vi "BusEvents.vi"(0 "EventArray":variant[](array[variant]), 7 "Error in":errorcluster[](array[cluster]), 10 "ModuleList":string[](array[string])) -> (20 "SyncEvts":T3, 21 "FGenEvts":T4, 22 "DigitizerEvts":T5, 23 "AnalysisBroadcastEvents":T2, 24 "SensorBdcstEvents":T1, 27 "Error out":errorcluster[](array[cluster]))   [LabVIEW 2014]
uses:
  Modules/Digitizer/DigitizerModule/Protected/Broadcasts/clBroadcastEvents.ctl
  Modules/Digitizer/DigitizerModule/Protected/clEventType.ctl
  Modules/FGen/FgenModule/Protected/Broadcasts/clBroadcastEvents.ctl
  Modules/FGen/FgenModule/Protected/clEventType.ctl
  Modules/Sync/SyncModule/Protected/Broadcasts/clBroadcastEvents.ctl
  Modules/Sync/SyncModule/Protected/clEventType.ctl
  Modules/Analysis/AnalysisModule/Protected/Broadcasts/clBroadcastEvents.ctl
  Modules/Analysis/AnalysisModule/Protected/clEventType.ctl
  Modules/Sensor/SensorModule/Protected/Broadcasts/clBroadcastEvents.ctl
  Modules/Sensor/SensorModule/Protected/clEventType.ctl
  <vilib>/Utility/error.llb/Error Cluster From Error Code.vi
  <vilib>/ErrorRing/Error Ring.xnode
  Modules/Digitizer/DigitizerModule/DigitizerModule.lvlib
  Modules/FGen/FgenModule/FgenModule.lvlib
  Modules/Sync/SyncModule/SyncModule.lvlib
  <userlib>/NIST/NISTErrorLib/NISTErrorLib.lvlib
  Modules/Analysis/AnalysisModule/AnalysisModule.lvlib
  Modules/Sensor/SensorModule/SensorModule.lvlib
panel:
  # "If you want to add other Broadcast Events, open this typedef, copy an existing event and rename it to your event name.\n\nNext create an \"arg\" typedef for the  data and put it into PublicAPI/Arguments/Broadcasts\n\nAfter that, you will need to create a new roadcast vi in Protected/Broadcast.  Look at DidInit.vi or the reportError.vi as examples."
  # "If you want to add other Broadcast Events, open this typedef, copy an existing event and rename it to your event name.\n\nNext create an \"arg\" typedef for the  data and put it into PublicAPI/Arguments/Broadcasts\n\nAfter that, you will need to create a new roadcast vi in Protected/Broadcast.  Look at DidInit.vi or the reportError.vi as examples."
  # "If you want to add other Broadcast Events, open this typedef, copy an existing event and rename it to your event name.\n\nNext create an \"arg\" typedef for the  data and put it into PublicAPI/Arguments/Broadcasts\n\nAfter that, you will need to create a new roadcast vi in Protected/Broadcast.  Look at DidInit.vi or the reportError.vi as examples."
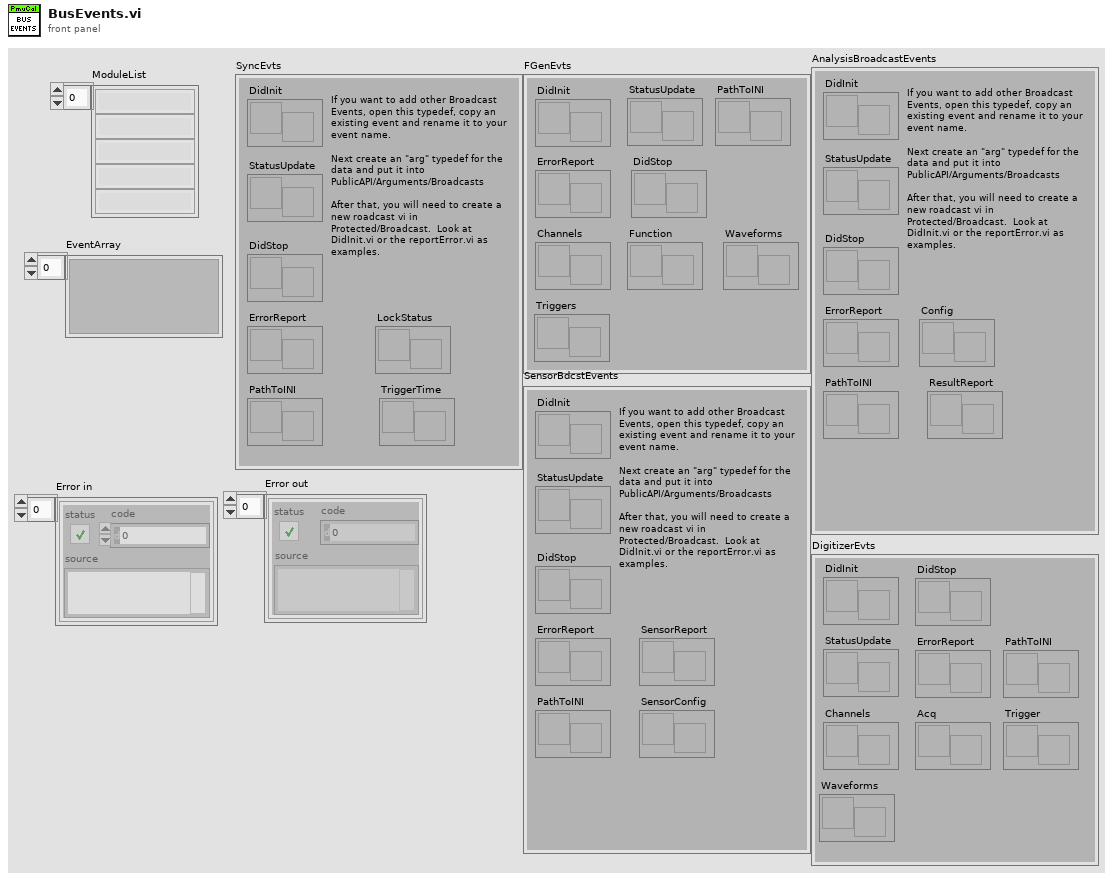
[diagram p1: front panel]
types:
  T1 = typedef "SensorModule.lvlib/clBroadcastEvents.ctl" = cluster{"DidInit":refnum<user-event>, "StatusUpdate":refnum<user-event>, "ErrorReport":refnum<user-event>, "DidStop":refnum<user-event>, "PathToINI":refnum<user-event>, "SensorReport":refnum<user-event>, "SensorConfig":refnum<user-event>}
  T2 = typedef "AnalysisModule.lvlib/clBroadcastEvents.ctl" = cluster{"DidInit":refnum<user-event>, "StatusUpdate":refnum<user-event>, "ErrorReport":refnum<user-event>, "DidStop":refnum<user-event>, "PathToINI":refnum<user-event>, "Config":refnum<user-event>, "ResultReport":refnum<user-event>}
  T3 = typedef "SyncModule.lvlib/clBroadcastEvents.ctl" = cluster{"DidInit":refnum<user-event>, "StatusUpdate":refnum<user-event>, "ErrorReport":refnum<user-event>, "DidStop":refnum<user-event>, "PathToINI":refnum<user-event>, "TriggerTime":refnum<user-event>, "LockStatus":refnum<user-event>}
  T4 = typedef "FgenModule.lvlib/clBroadcastEvents.ctl" = cluster{"DidInit":refnum<user-event>, "StatusUpdate":refnum<user-event>, "ErrorReport":refnum<user-event>, "DidStop":refnum<user-event>, "PathToINI":refnum<user-event>, "Channels":refnum<user-event>, "Function":refnum<user-event>, "Waveforms":refnum<user-event>, "Triggers":refnum<user-event>}
  T5 = typedef "DigitizerModule.lvlib/clBroadcastEvents.ctl" = cluster{"DidInit":refnum<user-event>, "StatusUpdate":refnum<user-event>, "ErrorReport":refnum<user-event>, "DidStop":refnum<user-event>, "PathToINI":refnum<user-event>, "Channels":refnum<user-event>, "Acq":refnum<user-event>, "Trigger":refnum<user-event>, "Waveforms":refnum<user-event>}
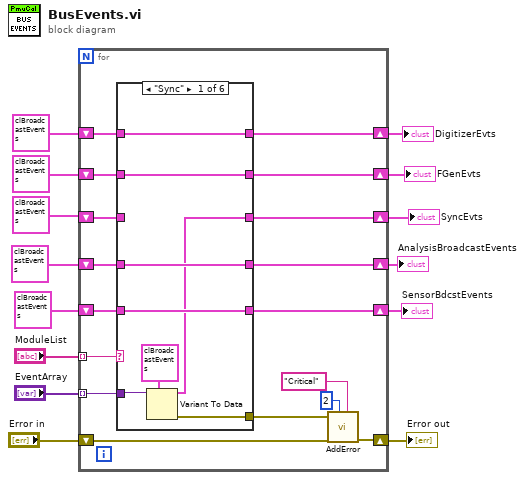
[diagram p0: block diagram]
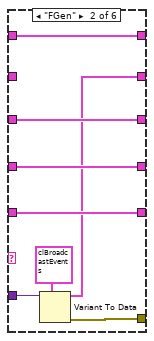
[diagram p2: hidden frame]
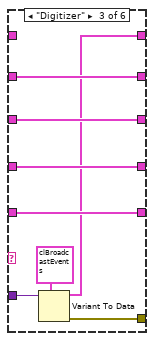
[diagram p3: hidden frame]
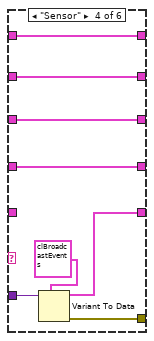
[diagram p4: hidden frame]
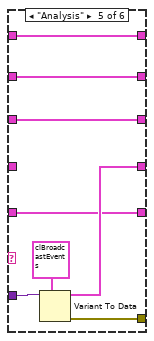
[diagram p5: hidden frame]
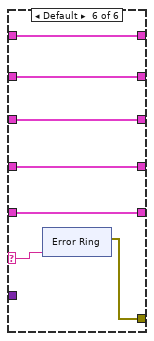
[diagram p6: hidden frame]
diagram:
  n1 = for {
    tunnel: "ModuleList" -> [w27] mode=indexing
    tunnel: "EventArray" -> [w26] mode=indexing
    shift-right: [w29] -> w5
    shift-left: "Error in" -> [w28]
    shift-right: [w23] -> w8
    shift-left: T5 {"DidInit"=refnum, "StatusUpdate"=refnum, "ErrorReport"=refnum, "DidStop"=refnum, "PathToINI"=refnum, "Channels"=refnum, "Acq"=refnum, "Trigger"=refnum, "Waveforms"=refnum} ("clBroadcastEvents") -> [w24]
    shift-right: [w19] -> w6
    shift-left: T3 {"DidInit"=refnum, "StatusUpdate"=refnum, "ErrorReport"=refnum, "DidStop"=refnum, "PathToINI"=refnum, "TriggerTime"=refnum, "LockStatus"=refnum} ("SyncBroadcastEvents") -> [w21]
    shift-right: [w20] -> w7
    shift-left: T4 {"DidInit"=refnum, "StatusUpdate"=refnum, "ErrorReport"=refnum, "DidStop"=refnum, "PathToINI"=refnum, "Channels"=refnum, "Function"=refnum, "Waveforms"=refnum, "Triggers"=refnum} ("clBroadcastEvents") -> [w22]
    shift-right: [w17] -> w3
    shift-left: T2 {"DidInit"=refnum, "StatusUpdate"=refnum, "ErrorReport"=refnum, "DidStop"=refnum, "PathToINI"=refnum, "Config"=refnum, "ResultReport"=refnum} ("AnalysisBroadcastEvents") -> [w18]
    shift-right: [w15] -> w1
    shift-left: T1 {"DidInit"=refnum, "StatusUpdate"=refnum, "ErrorReport"=refnum, "DidStop"=refnum, "PathToINI"=refnum, "SensorReport"=refnum, "SensorConfig"=refnum} ("SensorBdcstEvents") -> [w16]
    n2 = case shown="\"Sync\"" w27 {
      selector: w27 -> [_ _ _ _ _ w75]
      tunnel: w26 -> [w38 w47 w51 w60 w71 _]
      tunnel: [w37 w46 w55 w63 w70 w74] -> w25
      tunnel: w24 -> [w35 w44 _ w58 w67 w78]
      tunnel: [w35 w44 w48 w58 w67 w78] -> w23
      tunnel: w22 -> [w36 _ w53 w62 w66 w77]
      tunnel: [w36 w40 w53 w62 w66 w77] -> w20
      tunnel: w21 -> [_ w43 w52 w61 w65 w76]
      tunnel: [w32 w43 w52 w61 w65 w76] -> w19
      tunnel: [w34 w42 w50 w59 w68 w73] -> w17
      tunnel: w18 -> [w34 w42 w50 w59 _ w73]
      tunnel: [w33 w41 w49 w56 w64 w72] -> w15
      tunnel: w16 -> [w33 w41 w49 _ w64 w72]
      frame "Sync" {
        n3 = Variant To Data(type=T3 {"DidInit"=refnum, "StatusUpdate"=refnum, "ErrorReport"=refnum, "DidStop"=refnum, "PathToINI"=refnum, "TriggerTime"=refnum, "LockStatus"=refnum} ("SyncBroadcastEvents"), Variant=w38) -> (data=w32:T3, error out=w37:errorcluster)  [unwired: 1 in]
      }
      frame "FGen" {
        n4 = Variant To Data(type=T4 {"DidInit"=refnum, "StatusUpdate"=refnum, "ErrorReport"=refnum, "DidStop"=refnum, "PathToINI"=refnum, "Channels"=refnum, "Function"=refnum, "Waveforms"=refnum, "Triggers"=refnum} ("clBroadcastEvents"), Variant=w47) -> (data=w40:T4, error out=w46:errorcluster)  [unwired: 1 in]
      }
      frame "Digitizer" {
        n5 = Variant To Data(type=T5 {"DidInit"=refnum, "StatusUpdate"=refnum, "ErrorReport"=refnum, "DidStop"=refnum, "PathToINI"=refnum, "Channels"=refnum, "Acq"=refnum, "Trigger"=refnum, "Waveforms"=refnum} ("clBroadcastEvents"), Variant=w51) -> (data=w48:T5, error out=w55:errorcluster)  [unwired: 1 in]
      }
      frame "Sensor" {
        n6 = Variant To Data(type=T1 {"DidInit"=refnum, "StatusUpdate"=refnum, "ErrorReport"=refnum, "DidStop"=refnum, "PathToINI"=refnum, "SensorReport"=refnum, "SensorConfig"=refnum} ("SensorBdcstEvents"), Variant=w60) -> (data=w56:T1, error out=w63:errorcluster)  [unwired: 1 in]
      }
      frame "Analysis" {
        n7 = Variant To Data(type=T2 {"DidInit"=refnum, "StatusUpdate"=refnum, "ErrorReport"=refnum, "DidStop"=refnum, "PathToINI"=refnum, "Config"=refnum, "ResultReport"=refnum} ("AnalysisBroadcastEvents"), Variant=w71) -> (data=w68:T2, error out=w70:errorcluster)  [unwired: 1 in]
      }
      frame Default {
        n8 = xnode "Error Ring"("parameter 0"=w75) -> ("error out"=w74:errorcluster)
      }
    }
    n9 = call <userlib>:"AddError.vi"("Severity"="Critical", "Priority"=u8 2, "ErrorArray"=w28, "error in (no error)"=w25) -> ("ErrorArray"=w29:errorcluster[])  [unwired: 6 in, 1 out]
  }
  "Error out" <- w5
  "DigitizerEvts" <- w8
  "FGenEvts" <- w7
  "SyncEvts" <- w6
  "AnalysisBroadcastEvents" <- w3
  "SensorBdcstEvents" <- w1
